vi "From TCP Ref.vi"(8 "error in (no error)":errorcluster, 11 "TCP Connection":refnum<k5>) -> (0 "error out":errorcluster, 3 "TCPStream out":refnum<class "TCPStream.lvclass">)   [LabVIEW 2020, in "HTTP Utils.lvlib" / "TCPStream.lvclass"]
uses:
  TCPStream.lvclass
  C:/Program Files (x86)/National Instruments/LabVIEW 2020/vi.lib/IlluminatedG/lv-stream/stream/Stream.lvclass
  TCPStream.lvclass/TCPStream.ctl
  <vilib>/IlluminatedG/lv-stream/stream/Stream.lvclass
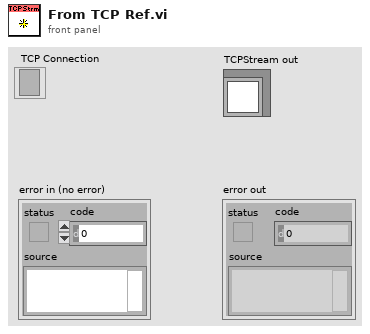
[diagram p1: front panel]
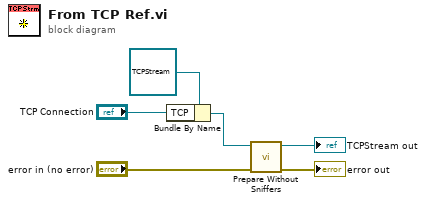
[diagram p0: block diagram]
diagram:
  n1 = Bundle By Name(cluster=refnum<class "TCPStream.lvclass"> refnum ("TCPStream in"), "TCP"="TCP Connection") -> (w1:refnum<class "TCPStream.lvclass">)
  n2 = call <vilib>:"Prepare Without Sniffers.vi"("error in (no error)"="error in (no error)", "Stream in"=w1) -> ("error out"=→"error out":errorcluster, "Stream out"=→"TCPStream out":refnum<class "TCPStream.lvclass">)  [unwired: 8 in]
